vi "Nullkoeffizienten entfernen IAG.vi"(9 "threshold type":T1 caption="Schwellwerttyp" items=["Absoluter Wert", "Relativer Wert"], 10 "threshold":dbl caption="Schwellwert", 11 "P(x) In":dbl[](array[numeric]) caption="P(x) (Eingang)" format="%#.6g") -> (2 "number of zero coefficients":i32 caption="Anzahl der Nullkoeffizienten", 3 "P(x) Out":dbl[](array[numeric]) caption="P(x) (Ausgang)" format="%#.6g")   [LabVIEW 2020, in "Linearisierung v2.lvlib"]
uses:
  Linearisierung v2.lvlib
  <vilib>/Analysis/polynomials.llb/Remove Zero Threshold Type.ctl
  <vilib>/Analysis/NI_AALPro.lvlib
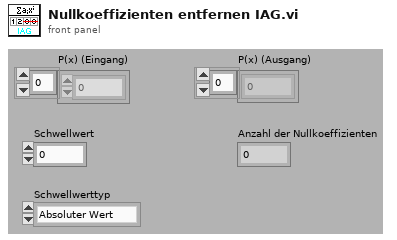
[diagram p1: front panel]
types:
  T1 = typedef "NI_AALPro.lvlib/Remove Zero Threshold Type.ctl" = u16
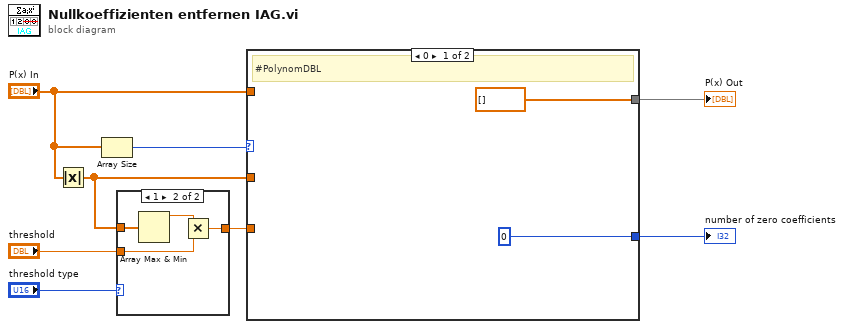
[diagram p0: block diagram]
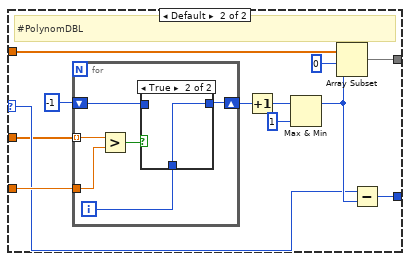
[diagram p3: hidden frame]
diagram:
  n1 = Absolute Value(x="P(x) In") -> (abs(x)=w8:dbl[])
  n2 = Array Size(array="P(x) In") -> (size(s)=w2:i32)
  n3 = case shown="1" "threshold type" {
    tunnel: "threshold" -> [w9 w11]
    tunnel: [w9 w10] -> w7
    tunnel: w8 -> [_ w13]
    frame 0, Default {
    }
    frame 1 {
      n4 = Array Max & Min(array=w13) -> (max value=w12:dbl)  [unwired: 3 out]
      n5 = Multiply(x=w12, y=w11) -> (x*y=w10:dbl)
    }
  }
  n6 = case shown="0" w2 {
    selector: w2 -> [_ w18]
    tunnel: [dbl[] [] ("BDL") w22] -> w1
    tunnel: "P(x) In" -> [_ w21]
    tunnel: w7 -> [_ w20]
    tunnel: [0 w17] -> w3
    tunnel: w8 -> [_ w16]
    frame 0 {
      # "#PolynomDBL"
    }
    frame Default {
      # "#PolynomDBL"
      n7 = for {
        shift-right: [w32] -> w26
        shift-left: -1 -> [w31]
        tunnel: w20 -> [w30]
        tunnel: w16 -> [w28] mode=indexing
        i -> [w33]
        n8 = Greater?(x=w28, y=w30) -> (0:w29:bool)
        n9 = case shown="True" w29 {
          tunnel: w33 -> [_ w35]
          tunnel: [w34 w35] -> w32
          tunnel: w31 -> [w34 _]
          frame False {
          }
          frame True {
          }
        }
      }
      n10 = Increment(x=w26) -> (x+1=w24:i32)
      n11 = Max & Min(x=w24, y=1) -> (max(x,y)=w19:i32)  [unwired: 1 out]
      n12 = Array Subset(array=w21, index=0, length=w19) -> (w22:dbl[])
      n13 = Subtract(x=w18, y=w19) -> (x-y=w17:i32)
    }
  }
  "P(x) Out" <- w1
  "number of zero coefficients" <- w3
